vi "Teleop.vi"(10 "Match Info":T1={"Autonomous Elapsed Seconds"=0.0, "TeleOp Elapsed Seconds"=0.0, "Disabled Elapsed Seconds"=0.0, "Visited Autonomous"=FALSE, "Visited TeleOp"=FALSE, "Visited Disabled"=FALSE, "Autonomous Settings"={"Autonomous Style"=enum."Independent", "VI Refnum"=refnum}}, 11 "Call Context":T2) -> ()   [LabVIEW 2016]
doc: "This VI is called for each TeleOp packet received from the DS where the robot is not disabled. It is often used to read from the joysticks and update I/O or to update setpoints for timed control loops. It should complete and return within 20 milliseconds or it may miss DS packets."
uses:
  <vilib>/Rock Robotics/WPI/DriverStation/WPI_DriverStationDerivedRobotMode.ctl
  <vilib>/Rock Robotics/WPI/DriverStation/WPI_DriverStationMatch Info.ctl
  <vilib>/Rock Robotics/WPI/ThirdParty/CanMotor/TalonSRX/WPI_CANTalonSRX_APIControlMode.ctl
  <vilib>/Rock Robotics/WPI/Relay/WPI_RelayValue.ctl
  <vilib>/Rock Robotics/WPI/Utilities/WPI_GetSetVariantRefNum.vi
  Robot Global Data.vi
  <vilib>/Rock Robotics/Network Tables/NT Read Number.vi
  <vilib>/Rock Robotics/Network Tables/NT Write Number.vi
  <vilib>/Rock Robotics/WPI/RobotDrive/WPI_RobotDriveMecanumDrive_Cartesian.vi
  <vilib>/Rock Robotics/Network Tables/NT Write Numeric Array.vi
panel:
  in  "LED Toggle":bool
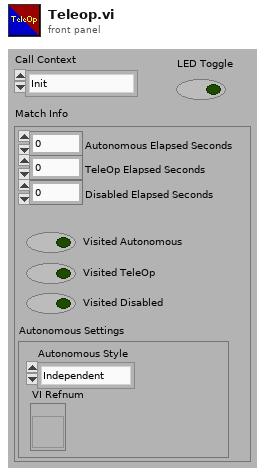
[diagram p1: front panel]
types:
  T1 = typedef "WPI_DriverStationMatch Info.ctl" = cluster{"Autonomous Elapsed Seconds":dbl, "TeleOp Elapsed Seconds":dbl, "Disabled Elapsed Seconds":dbl, "Visited Autonomous":bool, "Visited TeleOp":bool, "Visited Disabled":bool, "Autonomous Settings":cluster{"Autonomous Style":enum16{"Iterative", "Independent"}, "VI Refnum":refnum<vi>}}
  T2 = typedef "WPI_DriverStationDerivedRobotMode.ctl" = enum16{"Init", "Execute", "Stop"}
  T3 = typedef "WPI_CANTalonSRX_APIControlMode.ctl" = enum8{"Percent VBus", "Speed", "Position", "Slave", "Unchanged / Invalid", "Voltage Compensation", "Current", "Motion Profile", "Motion Magic"}
  T4 = typedef "WPI_JoystickDevRef.ctl" = cluster{"Device":T5}
  T5 = typedef "WPI_JoystickDeviceEnum.ctl" = enum16{"USB 0", "USB 1", "USB 2", "USB 3", "USB 4", "USB 5"}
  T6 = typedef "WPI_RelayDevRef.ctl" = cluster{"DevStatus":errorcluster, "Relay Channel":T7, "Relay Direction":T8}
  T7 = typedef "FPGA_DIORelayChannel.ctl" = enum8{"Relay 0", "Relay 1", "Relay 2", "Relay 3", "Invalid"}
  T8 = typedef "WPI_RelayDirection.ctl" = enum16{"Both directions", "Forward only", "Reverse only"}
  T9 = typedef "WPI_RelayValue.ctl" = enum16{"Off", "On", "Forward", "Reverse"}
  T10 = typedef "WPI_RobotDriveDevRef.ctl" = cluster{"DevStatus":errorcluster, "Motors[]":T11[], "Square Inputs":bool, "Max Output":dbl}
  T11 = typedef "WPI_MotorControlDeviceRef.ctl" = cluster{"DeviceStatus":errorcluster, "Type":T12, "PWM":cluster{"PWM Channel":T13, "DeadBand":T14}, "CAN":cluster{"Device Number":u8, "SetOutput VI Ref":variant, "GetOutput VI Ref":variant, "Enable VI Ref":variant, "Disable VI Ref":variant, "Data":variant}, "Invert":bool}
  T12 = typedef "WPI_MotorControlType.ctl" = enum16{"PWM", "CAN"}
  T13 = typedef "FPGA_DIOPWMChannel.ctl" = enum8{"PWM 0", "PWM 1", "PWM 2", "PWM 3", "PWM 4", "PWM 5", "PWM 6", "PWM 7", "PWM 8", "PWM 9", "PWM MXP 0", "PWM MXP 1", "PWM MXP 2", "PWM MXP 3", "PWM MXP 4", "PWM MXP 5", "PWM MXP 6", "PWM MXP 7", "PWM MXP 8", "PWM MXP 9", "Invalid"}
  T14 = typedef "WPI_PWMDeadband.ctl" = cluster{"Name":string, "maxPositivePwm":i32, "minPositivePwm":i32, "centerPwm":i32, "maxNegativePwm":i32, "minNegativePwm":i32, "angularRange":u16}
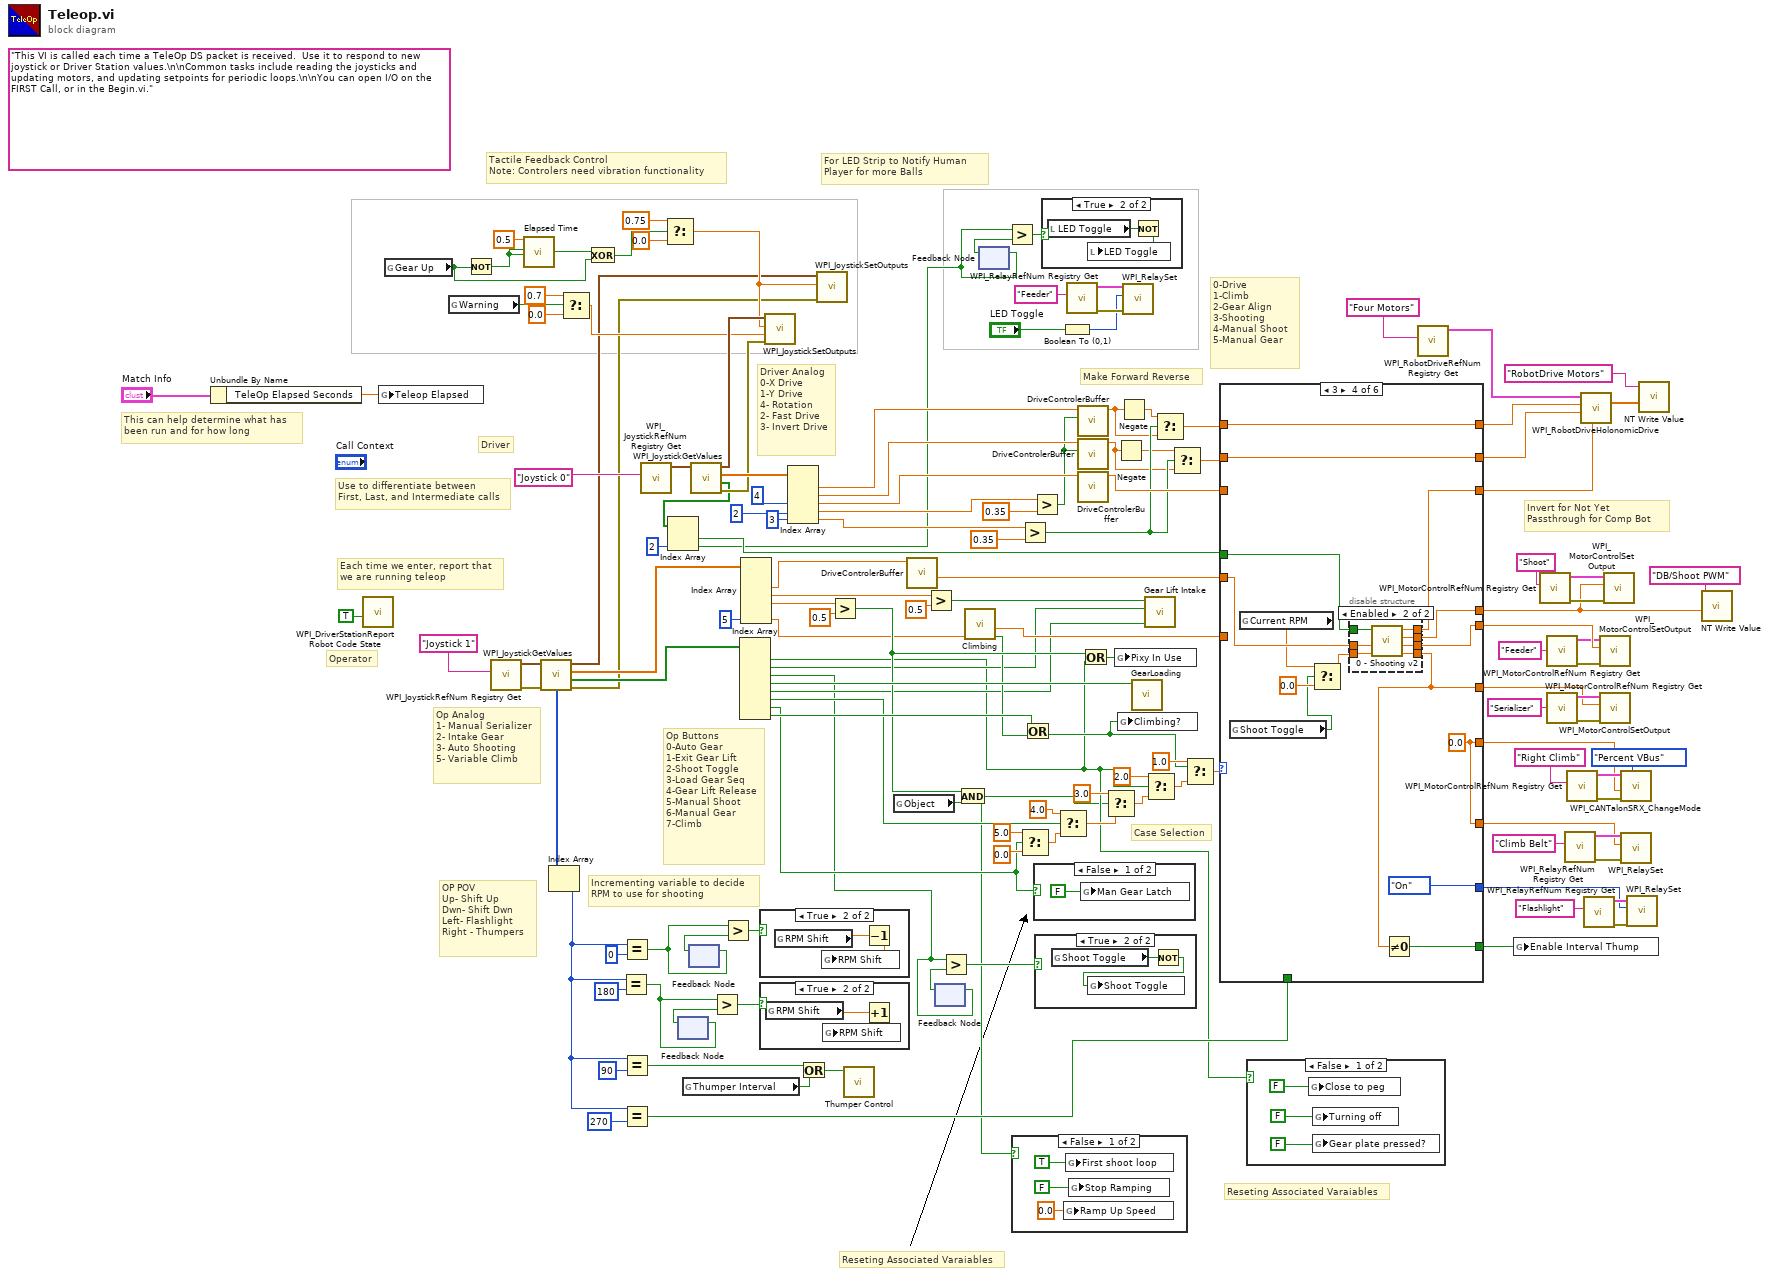
[diagram p0: block diagram]
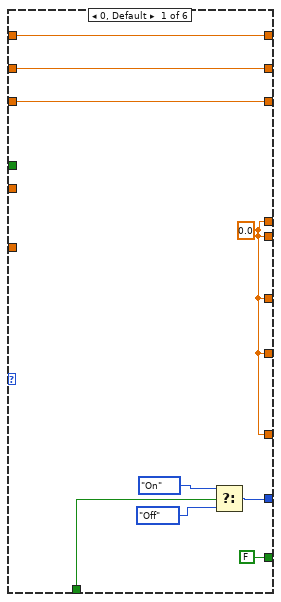
[diagram p9: hidden frame]
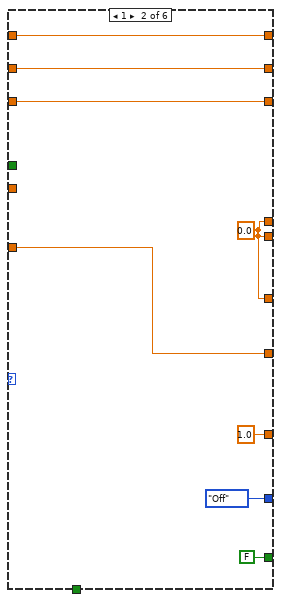
[diagram p10: hidden frame]
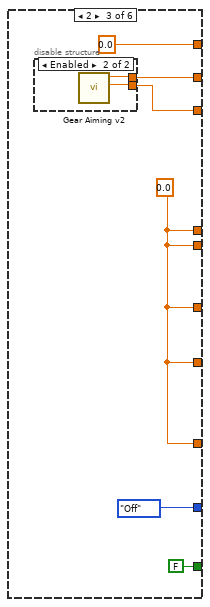
[diagram p11: hidden frame]
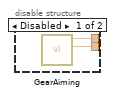
[diagram p12: hidden frame]
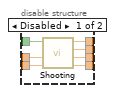
[diagram p13: hidden frame]
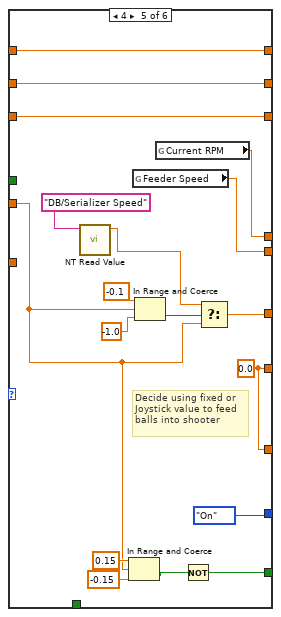
[diagram p14: hidden frame]
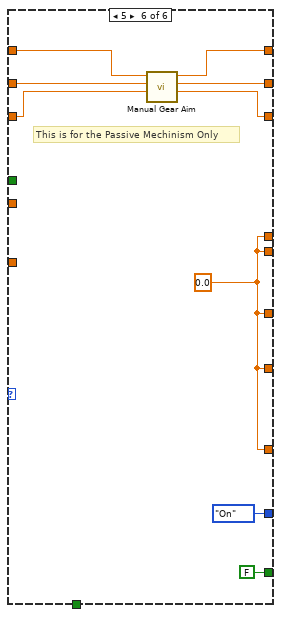
[diagram p15: hidden frame]
diagram:
  (unwired) "This VI is called each time a TeleOp DS packet is received.  Use it to respond to new joystick or Driver Station values.\n\nCommon tasks include reading the joysticks and updating motors, and updating setpoints for periodic loops.\n\nYou can open I/O on the FIRST Call, or in the Begin.vi."
  # "Reseting Associated Varaiables"
  # "Incrementing variable to decide\nRPM to use for shooting"
  # "Make Forward Reverse"
  # "Reseting Associated Varaiables"
  # "Case Selection"
  # "Driver"
  # "Operator"
  # "Tactile Feedback Control\nNote: Controlers need vibration functionality"
  # "For LED Strip to Notify Human \nPlayer for more Balls"
  # "OP POV \nUp- Shift Up\nDwn- Shift Dwn\nLeft- Flashlight\nRight - Thumpers"
  # "Invert for Not Yet\nPassthrough for Comp Bot"
  # "Op Analog\n1- Manual Serializer\n2- Intake Gear\n3- Auto Shooting\n5- Variable Climb"
  # "Op Buttons\n0-Auto Gear\n1-Exit Gear Lift\n2-Shoot Toggle\n3-Load Gear Seq\n4-Gear Lift Release\n5-Manual Shoot\n6-Manual Gear\n7-Climb"
  # "Driver Analog\n0-X Drive\n1-Y Drive\n4- Rotation\n2- Fast Drive\n3- Invert Drive"
  # "0-Drive\n1-Climb\n2-Gear Align\n3-Shooting\n4-Manual Shoot\n5-Manual Gear"
  # "Each time we enter, report that\nwe are running teleop"
  # "Use to differentiate between\nFirst, Last, and Intermediate calls"
  # "This can help determine what has\nbeen run and for how long"
  n1 = Unbundle By Name("Match Info") -> ("TeleOp Elapsed Seconds"=w67:dbl)
  n2 = call <vilib>:"WPI_DriverStationReport Robot Code State.vi"("TeleOp"=TRUE ("Autonomous")) -> ()  [unwired: 10 in, 1 out]
  n3 = global write "Robot Global Data.vi" "Teleop Elapsed"(w67) -> ()
  n4 = global read "Robot Global Data.vi" "Gear Up"() -> (w21:bool)
  n5 = global read "Robot Global Data.vi" "Warning"() -> (w55:bool)
  n6 = Not(x=w21) -> (.not. x?=w25:bool)
  n7 = call <vilib>:"WPI_JoystickRefNum Registry Get.vi"("refnum name"="Joystick 1") -> ("error out"=w27:errorcluster, "JoystickDevRef"=w121:T4)  [unwired: 1 in, 8 out]
  n8 = call "Elapsed Time"("Time Target (s)"=0.5, "Reset"=w25, "Auto Reset"=w25) -> ("Time has Elapsed"=w20:bool)  [unwired: 9 in, 7 out]
  n9 = call <vilib>:"WPI_JoystickGetValues.vi"("error in (no error)"=w27, "JoystickDevRef"=w121) -> ("error out"=w17:errorcluster, "Buttons"=w114:bool[], "Axes"=w102:dbl[], "JoystickDevRef"=w18:T4, "POVs"=w76:i16[])  [unwired: 5 in]
  n10 = Index Array(array=w76) -> (element=w40:i16)  [unwired: 1 in]
  n11 = Select(t=0.7, s=w55, f=0.0) -> (s? t:f=w45:dbl)
  n12 = Exclusive Or(1:w21, 2:w20) -> (0:w22:bool)
  n13 = Equal?(x=w40, y=i16 180) -> (x = y?=w68:bool)
  n14 = Equal?(x=w40, y=i16 0) -> (x = y?=w72:bool)
  n15 = Equal?(x=w40, y=i16 90) -> (x = y?=w33:bool)
  n16 = Equal?(x=w40, y=i16 270) -> (x = y?=w39:bool)
  n17 = call <vilib>:"WPI_JoystickRefNum Registry Get.vi"("refnum name"="Joystick 0") -> ("JoystickDevRef"=w140:T4)  [unwired: 1 in, 9 out]
  n18 = Select(t=0.75, s=w22, f=0.0) -> (s? t:f=w19:dbl)
  n19 = feedback #1() -> (w69:bool)  [unwired: 1 in]
  n20 = feedback-in #1(w68) -> ()
  n21 = global read "Robot Global Data.vi" "Thumper Interval"() -> (w32:bool)
  n22 = feedback-in #2(w72) -> ()
  n23 = feedback #2() -> (w71:bool)  [unwired: 1 in]
  n24 = call <vilib>:"WPI_JoystickGetValues.vi"("JoystickDevRef"=w140) -> ("error out"=w56:errorcluster, "Buttons"=w52:bool[], "Axes"=w138:dbl[], "JoystickDevRef"=w57:T4)  [unwired: 6 in, 1 out]
  n25 = Index Array(array=w52, index #2=2 ("index")) -> (element #1=w51:bool, element #2=w6:bool)  [unwired: 1 in]
  n26 = Greater?(x=w68, y=w69) -> (0:w70:bool)
  n27 = Greater?(x=w72, y=w71) -> (0:w73:bool)
  n28 = Index Array(array=w114) -> (element #1=w2:bool, element #2=w28:bool, element #3=w29:bool, element #4=w65:bool, element #5=w38:bool, element #6=w101:bool, element #7=w61:bool, element #8=w112:bool)  [unwired: 8 in]
  n29 = Index Array(array=w102, index #6=5 ("index")) -> (element #2=w98:dbl, element #3=w43:dbl, element #4=w100:dbl, element #6=w49:dbl)  [unwired: 5 in, 2 out]
  n30 = case shown="True" w73 {
    frame False {
    }
    frame True {
      n31 = global read "Robot Global Data.vi" "RPM Shift"() -> (w146:dbl)
      n32 = Decrement(x=w146) -> (x-1=w145:dbl)
      n33 = global write "Robot Global Data.vi" "RPM Shift"(w145) -> ()
    }
  }
  n34 = case shown="True" w70 {
    frame False {
    }
    frame True {
      n35 = global read "Robot Global Data.vi" "RPM Shift"() -> (w148:dbl)
      n36 = Increment(x=w148) -> (x+1=w147:dbl)
      n37 = global write "Robot Global Data.vi" "RPM Shift"(w147) -> ()
    }
  }
  n38 = call <vilib>:"WPI_JoystickSetOutputs.vi"("error in (no error)"=w56, "Right Rumble"=w45, "Left Rumble"=w19, "JoystickDevRef"=w57) -> ()  [unwired: 6 in, 2 out]
  n39 = Index Array(array=w138, index #3=4 ("index"), index #4=2 ("index"), index #5=3 ("index")) -> (element #1=w135:dbl, element #2=w134:dbl, element #3=w133:dbl, element #4=w119:dbl, element #5=w86:dbl)  [unwired: 2 in]
  n40 = Or(x=w33, y=w32) -> (x .or. y?=w35:bool)
  n41 = call <vilib>:"WPI_JoystickSetOutputs.vi"("error in (no error)"=w17, "Left Rumble"=w19, "JoystickDevRef"=w18) -> ()  [unwired: 7 in, 2 out]
  n42 = Greater?(x=w100, y=0.5) -> (0:w59:bool)
  n43 = call "Thumper Control.vi"("Thump"=w35) -> ()  [unwired: 11 in]
  n44 = global read "Robot Global Data.vi" "Object"() -> (w58:bool)
  n45 = call "DriveControlerBuffer.vi"("Input"=w98) -> ("Serializer Out"=w60:dbl)  [unwired: 9 in, 1 out]
  n46 = Greater?(x=w43, y=0.5) -> (0:w42:bool)
  n47 = feedback #3() -> (w31:bool)  [unwired: 1 in]
  n48 = feedback-in #3(w29) -> ()
  n49 = Greater?(x=w29, y=w31) -> (0:w30:bool)
  n50 = And(x=w59, y=w58) -> (x .and. y?=w1:bool)
  n51 = call "Climbing.vi"("Joystick In"=w49) -> ("Override"=w48:bool, "Climb Speed"=w47:dbl)  [unwired: 9 in]
  n52 = feedback #4() -> (w7:bool)  [unwired: 1 in]
  n53 = feedback-in #4(w6) -> ()
  n54 = Greater?(x=w6, y=w7) -> (0:w5:bool)
  n55 = case shown="False" w1 {
    frame False {
      n56 = global write "Robot Global Data.vi" "Ramp Up Speed"(0.0 ("Ramp Up Speed")) -> ()
      n57 = global write "Robot Global Data.vi" "First shoot loop"(TRUE ("Latch")) -> ()
      n58 = global write "Robot Global Data.vi" "Stop Ramping"(FALSE ("Latch")) -> ()
    }
    frame True {
    }
  }
  n59 = Greater?(x=w86, y=0.35) -> (0:w82:bool)
  n60 = Select(t=5.0, s=w61, f=0.0) -> (s? t:f=w63:dbl)
  n61 = Or(x=w112, y=w48) -> (x .or. y?=w16:bool)
  n62 = Greater?(x=w119, y=0.35) -> (0:w117:bool)
  n63 = case shown="False" w61 {
    frame False {
      n64 = global write "Robot Global Data.vi" "Man Gear Latch"(FALSE ("Latch")) -> ()
    }
    frame True {
    }
  }
  n65 = case shown="True" w30 {
    frame False {
    }
    frame True {
      n66 = global read "Robot Global Data.vi" "Shoot Toggle"() -> (w154:bool)
      n67 = Not(x=w154) -> (.not. x?=w153:bool)
      n68 = global write "Robot Global Data.vi" "Shoot Toggle"(w153) -> ()
    }
  }
  n69 = case shown="True" w5 {
    frame False {
    }
    frame True {
      n70 = local read "LED Toggle"() -> (w156:bool)
      n71 = Not(x=w156) -> (.not. x?=w155:bool)
      n72 = local write "LED Toggle"(w155) -> ()
    }
  }
  n73 = Select(t=4.0, s=w101, f=w63) -> (s? t:f=w116:dbl)
  n74 = Boolean To (0,1)(Boolean="LED Toggle") -> (0, 1=w4:i16)
  n75 = call <vilib>:"WPI_RelayRefNum Registry Get.vi"("refnum name"="Feeder") -> ("error out"=w10:errorcluster, "RelayDevRef"=w9:T6)  [unwired: 9 in]
  n76 = call "DriveControlerBuffer.vi"("Fast Drive"=w117, "Input"=w135) -> ("Drive Output"=w81:dbl)  [unwired: 8 in, 1 out]
  n77 = call "DriveControlerBuffer.vi"("Fast Drive"=w117, "Input"=w134) -> ("Drive Output"=w80:dbl)  [unwired: 8 in, 1 out]
  n78 = call "DriveControlerBuffer.vi"("Input"=w133) -> ("Drive Output"=w83:dbl)  [unwired: 9 in, 1 out]
  n79 = Or(x=w59, y=w2) -> (x .or. y?=w66:bool)
  n80 = Select(t=3.0, s=w1, f=w116) -> (s? t:f=w130:dbl)
  n81 = global write "Robot Global Data.vi" "Pixy In Use"(w66) -> ()
  n82 = Negate(x=w80) -> (-x=w78:dbl)
  n83 = global write "Robot Global Data.vi" "Climbing?"(w16) -> ()
  n84 = Negate(x=w81) -> (-x=w79:dbl)
  n85 = call <vilib>:"WPI_RelaySet.vi"("error in (no error)"=w10, "RelayValue"=w4, "RelayDevRef"=w9) -> ()  [unwired: 7 in, 2 out]
  n86 = call "GearLoading.vi"("Activate"=w65) -> ()  [unwired: 11 in]
  n87 = call "Gear Lift Intake.vi"("Release"=w38, "Exit Button"=w28, "Trigger"=w42) -> ()  [unwired: 9 in]
  n88 = Select(t=2.0, s=w2, f=w130) -> (s? t:f=w131:dbl)
  n89 = Select(t=w79, s=w82, f=w81) -> (s? t:f=w85:dbl)
  n90 = Select(t=w78, s=w82, f=w80) -> (s? t:f=w84:dbl)
  n91 = Select(t=1.0, s=w16, f=w131) -> (s? t:f=w132:dbl)
  n92 = case shown="3" w132 {
    tunnel: [w165 w173 0.0 ("Output") w195 w230 w239] -> w126
    tunnel: w85 -> [w165 w173 _ w195 w230 w238]
    tunnel: [w164 w172 w178 w194 w229 w237] -> w123
    tunnel: w84 -> [w164 w172 _ w194 w229 w236]
    tunnel: [w163 w171 w177 w192 w228 w235] -> w125
    tunnel: w83 -> [w163 w171 _ _ w228 w234]
    tunnel: [w159 w170 w175 w198 w225 w233] -> w37
    tunnel: [w159 w170 w175 w191 w213 w233] -> w15
    tunnel: [w159 w167 w175 w196 w226 w233] -> w107
    tunnel: [w159 w170 w175 w185 w218 w233] -> w104
    tunnel: w60 -> [_ _ _ w193 w214 _]
    tunnel: [w161 WPI_RelayValue."Off" ("RelayValue") WPI_RelayValue."Off" ("RelayValue") WPI_RelayValue."On" ("RelayValue") WPI_RelayValue."On" ("RelayValue") WPI_RelayValue."On" ("RelayValue")] -> w95
    tunnel: [w159 1.0 ("Shooter Output") w175 w196 w226 w233] -> w90
    tunnel: w51 -> [_ _ _ w190 _ _]
    tunnel: w47 -> [_ w167 _ _ _ _]
    tunnel: w39 -> [w158 _ _ _ _ _]
    tunnel: [FALSE ("Thumper Out") FALSE ("Thumper Out") FALSE ("Thumper Out") w186 w215 FALSE ("Thumper Out")] -> w34
    frame 0, Default {
      w159 = 0.0 ("Shooter Output")
      n93 = Select(t=WPI_RelayValue."On", s=w158, f=WPI_RelayValue."Off" ("RelayValue")) -> (s? t:f=w161:T9)
    }
    frame 1 {
      w170 = 0.0 ("Shooter Output")
    }
    frame 2 {
      w175 = 0.0 ("Shooter Output")
      n94 = disable-structure shown="Enabled" {
        disable-tunnel: [w181 w183] -> w178
        disable-tunnel: [w180 w182] -> w177
        frame Disabled {
          n95 = call "GearAiming.vi"() -> ("Drive Rotate"=w180:dbl, "Drive Y"=w181:dbl)  [unwired: 10 in]
        }
        frame Enabled {
          n96 = call "Gear Aiming v2.vi"() -> ("Drive Rotate"=w182:dbl, "Drive Y"=w183:dbl)  [unwired: 10 in]
        }
      }
    }
    frame 3 {
      w196 = 0.0 ("Shooter Output")
      n97 = global read "Robot Global Data.vi" "Shoot Toggle"() -> (w187:bool)
      n98 = global read "Robot Global Data.vi" "Current RPM"() -> (w184:dbl)
      n99 = Select(t=w184, s=w187, f=0.0) -> (s? t:f=w189:dbl)
      n100 = disable-structure shown="Enabled" {
        disable-tunnel: [w205 w207] -> w198
        disable-tunnel: w193 -> [w204 w211]
        disable-tunnel: [w203 w206] -> w192
        disable-tunnel: [w202 w208] -> w191
        disable-tunnel: w190 -> [w201 w212]
        disable-tunnel: w189 -> [w200 w210]
        disable-tunnel: [w199 w209] -> w185
        frame Disabled {
          n101 = call "Shooting.vi"("Shoot override"=w200, "Serializer Override"=w204, "Lock PWM"=w201) -> ("Serializer Output"=w199:dbl, "Feeder Output"=w202:dbl, "Shooter PWM"=w205:dbl, "Rotation Out"=w203:dbl)  [unwired: 3 in]
        }
        frame Enabled {
          n102 = call "0 - Shooting v2.vi"("Shoot Override"=w210, "Serializer Override"=w211, "Lock PWM"=w212) -> ("Serializer Output"=w209:dbl, "Feeder Output"=w208:dbl, "Shooter PWM"=w207:dbl, "Rotation Out"=w206:dbl)  [unwired: 5 in]
        }
      }
      n103 = Not Equal To 0?(x=w185) -> (x != 0?=w186:bool)
    }
    frame 4 {
      w226 = 0.0 ("Shooter Output")
      # "Decide using fixed or\nJoystick value to feed\nballs into shooter"
      n104 = call-poly <vilib>:"NT Read Value.vi"("Name"="DB/Serializer Speed") -> ("Numeric"=w221:dbl)  [unwired: 9 in, 1 out]
      n105 = In Range and Coerce(upper limit=0.15, x=w214, lower limit=-0.15) -> (In Range?=w219:bool)  [unwired: 1 out]
      n106 = global read "Robot Global Data.vi" "Feeder Speed"() -> (w213:dbl)
      n107 = In Range and Coerce(upper limit=-0.1, x=w214, lower limit=-1.0) -> (In Range?=w220:bool)  [unwired: 1 out]
      n108 = global read "Robot Global Data.vi" "Current RPM"() -> (w225:dbl)
      n109 = Not(x=w219) -> (.not. x?=w215:bool)
      n110 = Select(t=w221, s=w220, f=w214) -> (s? t:f=w218:dbl)
    }
    frame 5 {
      w233 = 0.0
      # "This is for the Passive Mechinism Only"
      n111 = call "Manual Gear Aim.vi"("Rotate In"=w234, "Y In"=w236, "X Input"=w238) -> ("Rotate Out"=w235:dbl, "Y Out"=w237:dbl, "X Out"=w239:dbl)  [unwired: 6 in]
    }
  }
  n112 = case shown="False" w2 {
    frame False {
      n113 = global write "Robot Global Data.vi" "Close to peg"(FALSE ("Latch")) -> ()
      n114 = global write "Robot Global Data.vi" "Turning off"(FALSE ("Latch")) -> ()
      n115 = global write "Robot Global Data.vi" "Gear plate pressed?"(FALSE) -> ()
    }
    frame True {
    }
  }
  n116 = call <vilib>:"WPI_RobotDriveRefNum Registry Get.vi"("refnum name"="Four Motors") -> ("RobotDriveDevRef"=w142:T10)  [unwired: 1 in, 9 out]
  n117 = global write "Robot Global Data.vi" "Enable Interval Thump"(w34) -> ()
  n118 = call <vilib>:"WPI_MotorControlRefNum Registry Get.vi"("refnum name"="Shoot") -> ("error out"=w77:errorcluster, "MotorControlDevRef"=w89:T11)  [unwired: 9 in]
  n119 = call <vilib>:"WPI_MotorControlRefNum Registry Get.vi"("refnum name"="Feeder") -> ("error out"=w12:errorcluster, "MotorControlDevRef"=w14:T11)  [unwired: 9 in]
  n120 = call <vilib>:"WPI_MotorControlRefNum Registry Get.vi"("refnum name"="Serializer") -> ("error out"=w106:errorcluster, "MotorControlDevRef"=w105:T11)  [unwired: 9 in]
  n121 = call <vilib>:"WPI_RelayRefNum Registry Get.vi"("refnum name"="Climb Belt") -> ("error out"=w93:errorcluster, "RelayDevRef"=w92:T6)  [unwired: 9 in]
  n122 = call <vilib>:"WPI_MotorControlRefNum Registry Get.vi"("refnum name"="Right Climb") -> ("error out"=w110:errorcluster, "MotorControlDevRef"=w109:T11)  [unwired: 9 in]
  n123 = call-poly <vilib>:"WPI_RobotDriveHolonomicDrive.vi"("Rotation"=w125, "Y"=w123, "X"=w126, "RobotDriveDevRef"=w142) -> ("Motor Values"=w136:dbl[])  [unwired: 5 in, 2 out]
  n124 = call <vilib>:"WPI_RelayRefNum Registry Get.vi"("refnum name"="Flashlight") -> ("error out"=w96:errorcluster, "RelayDevRef"=w97:T6)  [unwired: 9 in]
  n125 = call <vilib>:"WPI_MotorControlSetOutput.vi"("error in (no error)"=w12, "Output"=w15, "MotorControlDevRef"=w14) -> ()  [unwired: 6 in, 3 out]
  n126 = call <vilib>:"WPI_MotorControlSetOutput.vi"("error in (no error)"=w106, "Output"=w104, "MotorControlDevRef"=w105) -> ()  [unwired: 6 in, 3 out]
  n127 = call <vilib>:"WPI_MotorControlSetOutput.vi"("error in (no error)"=w77, "Output"=w37, "MotorControlDevRef"=w89) -> ()  [unwired: 6 in, 3 out]
  n128 = call <vilib>:"WPI_CANTalonSRX_ChangeMode.vi"("error in (no error)"=w110, "Output"=w107, "Control Mode"=WPI_CANTalonSRX_APIControlMode."Percent VBus", "CAN Talon SRX Ref"=w109) -> ()  [unwired: 6 in, 2 out]
  n129 = call <vilib>:"WPI_RelaySet.vi"("error in (no error)"=w93, "RelayValue"=w90, "RelayDevRef"=w92) -> ()  [unwired: 7 in, 2 out]
  n130 = call <vilib>:"WPI_RelaySet.vi"("error in (no error)"=w96, "RelayValue"=w95, "RelayDevRef"=w97) -> ()  [unwired: 7 in, 2 out]
  n131 = call-poly <vilib>:"NT Write Value.vi"("Numeric Array"=w136, "Name"="RobotDrive Motors") -> ()  [unwired: 9 in, 1 out]
  n132 = call-poly <vilib>:"NT Write Value.vi"("Numeric"=w37, "Name"="DB/Shoot PWM") -> ()  [unwired: 9 in, 1 out]
